vi "_rep_cap_pack.vi"(3 "RepCapName CmdValues":string[](array[string]), 5 "RepCapName IDs":string[](array[string])) -> (0 "RepCap Type out":T1, 2 "RepCap IDs out":variant)   [LabVIEW 2022 SP3, in "hmp4000_rsidr_core.lvlib"]
uses:
  hmp4000_rsidr_core.lvlib
  _type_RepCap_Type.ctl
  whitespace.ctl
  Trim Whitespace One-Sided.vi
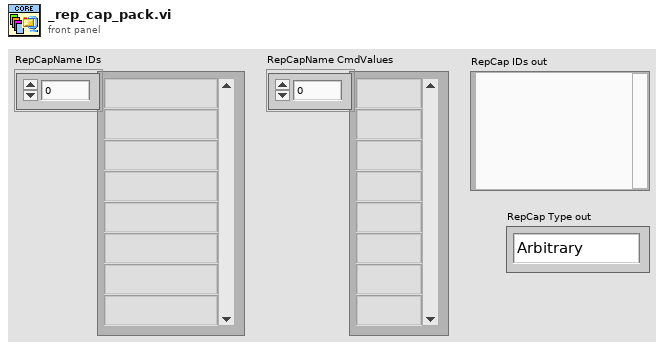
[diagram p1: front panel]
types:
  T1 = typedef "hmp4000_rsidr_core.lvlib/_type_RepCap_Type.ctl" = enum16{"Arbitrary", "SequentialNull", "Sequential"}
  T2 = typedef "whitespace.ctl" = u16
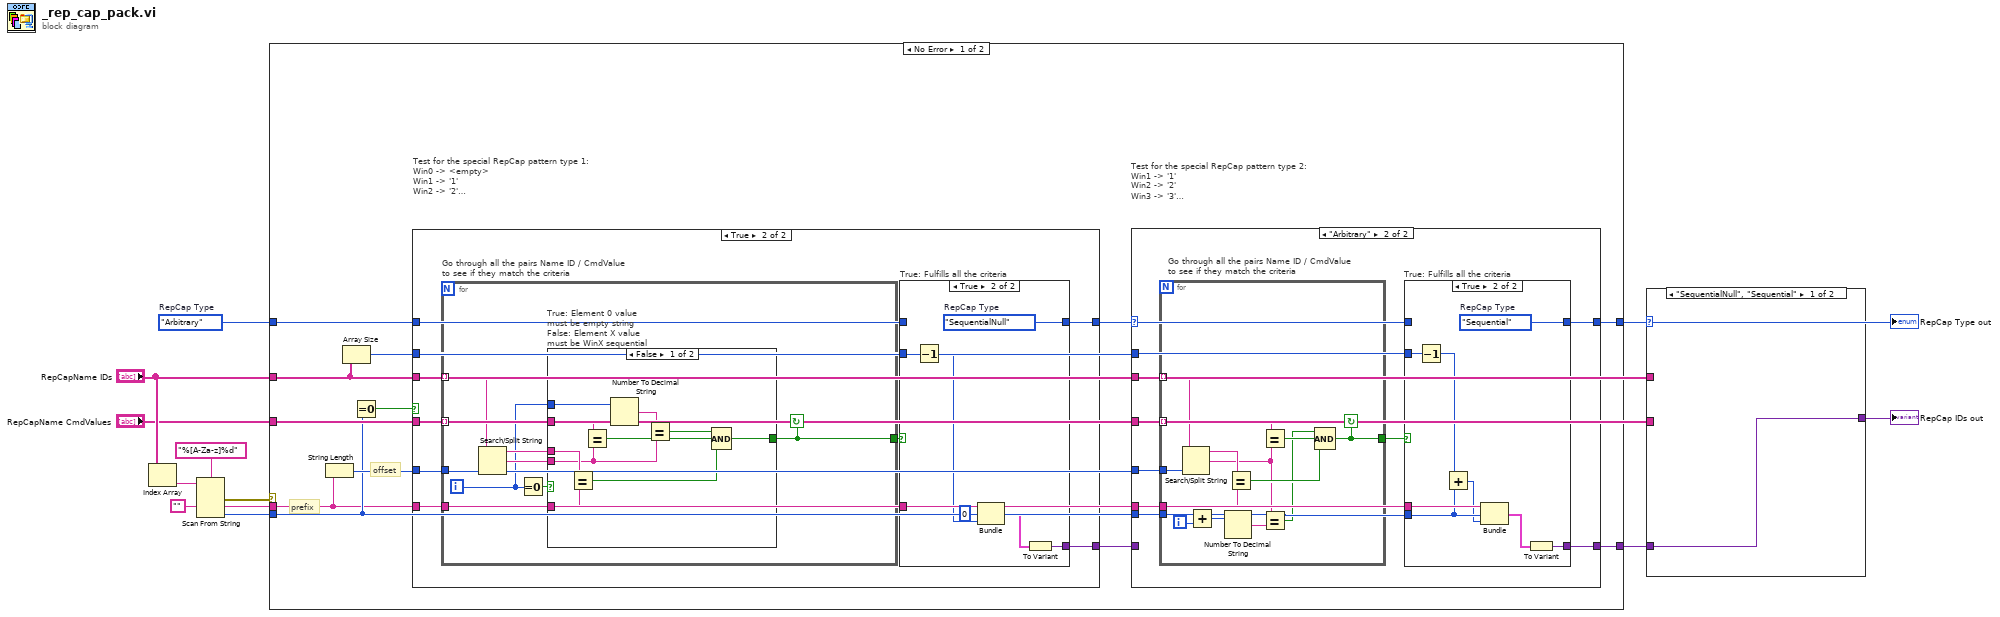
[diagram p0: block diagram]
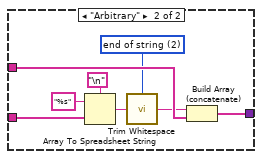
[diagram p2: hidden frame]
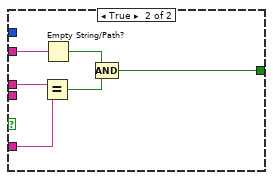
[diagram p7: hidden frame]
diagram:
  w1 = _type_RepCap_Type."Arbitrary"  # RepCap Type
  n1 = Index Array(array="RepCapName IDs") -> (element=w12:string)  [unwired: 1 in]
  n2 = Scan From String(format string="%[A-Za-z]%d" ("string"), input string=w12, default 1="" ("Empty String Constant")) -> (error out=w10:errorcluster, output 1=w5:string, output 2=w4:i32)  [unwired: 3 in, 2 out]
  n3 = case shown="No Error" w10 {
    tunnel: "RepCapName IDs" -> [w17 _]
    tunnel: "RepCapName CmdValues" -> [w22 _]
    tunnel: w5 -> [w19 _]
    tunnel: w4 -> [w20 _]
    tunnel: w1 -> [w23 w103]
    tunnel: [w15 w103] -> w2
    tunnel: [w14 _] -> w3
    frame No Error {
      # "offset"
      # "prefix"
      n4 = String Length(string=w19) -> (length=w21:i32)
      n5 = Array Size(array=w17) -> (size(s)=w16:i32)
      n6 = Equal To 0?(x=w20) -> (x = 0?=w24:bool)
      n7 = case "Test for the special RepCap pattern type 1:\nWin0 -> <empty>\nWin1 -> '1'\nWin2 -> '2'\n\nName IDs must start with Win0 and the first CmdValue must be empty\nFor all the further NameIDs WinX the value must be X\nX values must be sequential, without an interruption" shown="True" w24 {
        tunnel: w17 -> [_ w69]
        tunnel: w22 -> [_ w68]
        tunnel: w23 -> [w60 w64]
        tunnel: w21 -> [_ w67]
        tunnel: [w60 w63] -> w13
        tunnel: w19 -> [_ w65]
        tunnel: [_ w62] -> w18
        tunnel: w16 -> [_ w61]
        frame False {
        }
        frame True {
          n8 = for "Go through all the pairs Name ID / CmdValue\nto see if they match the criteria" {
            tunnel: w69 -> [w83] mode=indexing
            tunnel: w68 -> [w86] mode=indexing
            tunnel: w65 -> [w84]
            tunnel: w67 -> [w82]
            tunnel: [w79] -> w66
            i -> [w78]
            stop <- w79 continue-if-true
            n9 = Search/Split String(string=w83, offset (0)=w82) -> (substring before match=w81:string, match + rest of string=w80:string)  [unwired: 1 in, 1 out]
            n10 = Equal To 0?(x=w78) -> (x = 0?=w85:bool)
            n11 = case "True: Element 0 value must be empty string\nFalse: Element X value must be WinX sequential" shown="False" w85 {
              tunnel: w86 -> [w95 w102]
              tunnel: w84 -> [w96 w100]
              tunnel: w78 -> [w92 _]
              tunnel: w81 -> [w90 w101]
              tunnel: w80 -> [w89 _]
              tunnel: [w87 w97] -> w79
              frame False {
                n12 = Equal?(x=w90, y=w96) -> (x = y?=w94:bool)
                n13 = Equal?(x=w95, y=w89) -> (x = y?=w93:bool)
                n14 = Number To Decimal String(number=w92) -> (decimal integer string=w91:string)  [unwired: 1 in]
                n15 = Equal?(x=w91, y=w89) -> (x = y?=w88:bool)
                n16 = Compound Arithmetic op=AND(w88, w93, w94) -> (w87:bool)
              }
              frame True {
                n17 = Equal?(x=w101, y=w100) -> (x = y?=w99:bool)
                n18 = Empty String/Path?(string/path=w102) -> (empty?=w98:bool)
                n19 = Compound Arithmetic op=AND(w98, w99) -> (w97:bool)
              }
            }
          }
          n20 = case "True: Fulfills all the criteria" shown="True" w66 {
            tunnel: w65 -> [_ w77]
            tunnel: w64 -> [w70 _]
            tunnel: [w70 w71] -> w63
            tunnel: [_ w76] -> w62
            tunnel: w61 -> [_ w72]
            frame False {
            }
            frame True {
              w71 = _type_RepCap_Type."SequentialNull"  # RepCap Type
              n21 = Decrement(x=w72) -> (x-1=w73:i32)
              n22 = Bundle(w77, 0, w73) -> (w75:cluster{string, i32, i32})  [unwired: 1 in]
              n23 = To Variant(anything=w75) -> (Variant=w76:variant)
            }
          }
        }
      }
      n24 = case "Test for the special RepCap pattern type 2:\nWin1 -> '1'\nWin2 -> '2'\nWin3 -> '3'\n\nFor all the NameIDs WinX the value must be X\nX values must be sequential, without an interruption" shown="\"Arbitrary\"" w13 {
        selector: w13 -> [w25 w27]
        tunnel: w17 -> [_ w36]
        tunnel: w22 -> [_ w35]
        tunnel: w19 -> [_ w32]
        tunnel: w21 -> [_ w34]
        tunnel: [w25 w28] -> w15
        tunnel: w20 -> [_ w30]
        tunnel: w18 -> [w26 _]
        tunnel: [w26 w29] -> w14
        tunnel: w16 -> [_ w31]
        frame "SequentialNull", "Sequential" {
        }
        frame "Arbitrary" {
          n25 = for "Go through all the pairs Name ID / CmdValue\nto see if they match the criteria" {
            tunnel: w36 -> [w57] mode=indexing
            tunnel: w35 -> [w59] mode=indexing
            tunnel: w32 -> [w58]
            tunnel: w34 -> [w56]
            tunnel: [w54] -> w33
            tunnel: w30 -> [w50]
            i -> [w49]
            stop <- w54 continue-if-true
            n26 = Search/Split String(string=w57, offset (0)=w56) -> (substring before match=w55:string, match + rest of string=w47:string)  [unwired: 1 in, 1 out]
            n27 = Add(x=w50, y=w49) -> (x+y=w46:i32)
            n28 = Number To Decimal String(number=w46) -> (decimal integer string=w48:string)  [unwired: 1 in]
            n29 = Equal?(x=w55, y=w58) -> (x = y?=w53:bool)
            n30 = Equal?(x=w59, y=w47) -> (x = y?=w52:bool)
            n31 = Equal?(x=w47, y=w48) -> (x = y?=w51:bool)
            n32 = Compound Arithmetic op=AND(w51, w52, w53) -> (w54:bool)
          }
          n33 = case "True: Fulfills all the criteria" shown="True" w33 {
            tunnel: w32 -> [_ w45]
            tunnel: [w37 w38] -> w28
            tunnel: [_ w44] -> w29
            tunnel: w31 -> [_ w42]
            tunnel: w30 -> [_ w41]
            tunnel: w27 -> [w37 _]
            frame False {
            }
            frame True {
              w38 = _type_RepCap_Type."Sequential"  # RepCap Type
              n34 = Decrement(x=w42) -> (x-1=w39:i32)
              n35 = Add(x=w39, y=w41) -> (x+y=w40:i32)
              n36 = Bundle(w45, w41, w40) -> (w43:cluster{string, i32, i32})  [unwired: 1 in]
              n37 = To Variant(anything=w43) -> (Variant=w44:variant)
            }
          }
        }
      }
    }
    frame Error {
    }
  }
  "RepCap Type out" <- w2
  n38 = case shown="\"SequentialNull\", \"Sequential\"" w2 {
    tunnel: w3 -> [w104 _]
    tunnel: "RepCapName IDs" -> [_ w108]
    tunnel: "RepCapName CmdValues" -> [_ w112]
    tunnel: [w104 w107] -> w6
    frame "SequentialNull", "Sequential" {
    }
    frame "Arbitrary" {
      w105 = T2 2 items=["both", "start of string", "end of string"] ("location (both)")
      n39 = Array To Spreadsheet String(delimiter (Tab)="\n" ("Line Feed Constant"), array=w112, 3:"%s" ("format string")) -> (spreadsheet string=w109:string)
      n40 = call "Trim Whitespace.vi"("string"=w109, "location (both)"=w105) -> ("trimmed string"=w106:string)
      n41 = Build Array (concatenate)(w106, w108) -> (w107:string[])
    }
  }
  "RepCap IDs out" <- w6
